vi "Read Description.vi"(11 "Condiment Decorator in":refnum<class "Condiment Decorator.lvclass">) -> (2 "Description":string)   [LabVIEW 2013, in "Condiment Decorator.lvclass"]
uses:
  Condiment Decorator.lvclass
  Condiment Decorator.lvclass/Condiment Decorator.ctl
  Abstract Beverage/Abstract Beverage.lvclass
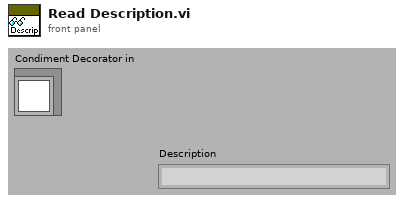
[diagram p1: front panel]
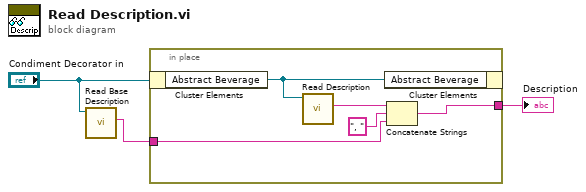
[diagram p0: block diagram]
diagram:
  n1 = call-dynamic "Read Base Description.vi"("Condiment Decorator in"="Condiment Decorator in") -> ("String"=w1:string)  [unwired: 10 in]
  n2 = in-place {
    in-place-border: [w7] -> w3
    in-place-border: w1 -> [w5]
    n3 = in-place-cluster #1("Condiment Decorator in") -> ("Abstract Beverage"=w6:refnum<class "Abstract Beverage.lvclass">)
    n4 = call-dynamic "Read Description.vi"("Abstract Beverage in"=w6) -> ("Description"=w8:string)  [unwired: 10 in]
    n5 = in-place-cluster #1("Abstract Beverage"=w6) -> ()  [unwired: 1 out]
    n6 = Concatenate Strings(w8, ", " ("string"), w5) -> (w7:string)
  }
  "Description" <- w3
